vi "FPGA Main.vi"() -> ()   [LabVIEW 2018]
doc: "This FPGA Main VI contains a control loop running in parallel with an RT watchdog loop.\n- The Control Loop performs control calculations on four input channels in parallel, and outputs the results to four output channels.\n- The RT Watchdog Loop checks for a periodic 'pet' from the RT Main VI to ensure communications between RT and FPGA are maintained."
uses:
  controls/Raw Values.ctl
  controls/FPGA State.ctl
  controls/Fill Valves.ctl
  controls/LNG PUGE.ctl
  controls/DECOUPLERS.ctl
  controls/VENT SYSTEM.ctl
  COMET  Extra Programs/controls/TTL Control.ctl
  controls/VENT SYSTEM INDICATORS.ctl
  controls/DECOUPLERS INDICATORS.ctl
  controls/FILL VALVES INDICATORS.ctl
  controls/LOX PURGE.ctl
  controls/LNG PURGE INDICATORS.ctl
  controls/LOX PURGE INDICATORS.ctl
  controls/IN TANK MEASUREMENTS.ctl
  controls/SYSTEM MEASUREMENTS.ctl
  Shared Variables/Flow Controller.ctl
  controls/FM Indicators.ctl
  <vilib>/Platform/TimedLoop/XDataNode/timing_clust.ctl
  <vilib>/Platform/TimedLoop/XDataNode/nitl_modes.ctl
  <vilib>/Platform/TimedLoop/XDataNode/wakeup.ctl
  <vilib>/rvi/FXPMathLib/basic elements/FxpIntAccumulator/subVIs/nifxpmath_IntAccumulator_SimConfig.ctl
  <vilib>/rvi/Emulation/niFpgaGetClockAttributes.vi
  <vilib>/rvi/Emulation/niFpgaSctlEmulationGetInTimedLoop.vi
  <vilib>/rvi/Emulation/niFpgaEmulationReportErrorSimple.vi
  <vilib>/rvi/eio/common/nirviEmuTemplateMethod_errors.vi
  <vilib>/rvi/Analysis/common/codeGenErrors/XNode/niFpgaXNodeCodeGenErrorHandle.vi
  <vilib>/rvi/Emulation/niFpgaCriticalErrorInLSC.vi
  <vilib>/rvi/FXPMathLib/basic elements/FxpIntAccumulator/simVIs/DllFxpIntAccumulator_sub.vi
  <vilib>/rvi/Emulation/niFpgaProcessEmulError.vi
  <vilib>/eio/EIONode/EIONode.xnode
  <vilib>/rvi/Analysis/measure/mean-var-std/XNode/niFpgaMean-Var-Std.xnode
  <vilib>/Platform/TimedLoop/XDataNode/XDataNode.xnode
  <vilib>/rvi/FXPMathLib/basic elements/FxpIntAccumulator/XNode/nifxpmath_IntAccumulator.xnode
  <vilib>/rvi/FXPMathLib/FxpMul/XNode/nifxpmath_Multiplier.xnode
  <vilib>/eio/EIOMethodNode/EIOMethodNode.xnode
  <vilib>/Platform/TimedLoop/XDataNode/XDNodeRunTimeDep.lvlib
  <vilib>/rvi/FXPMathLib/sim/FxpSim.dll
panel:
  out "Flow Controller 2":T1={"LOX_HE_MFC"=0.004, "LNG_HE_MFC"=0.004}
  out "FM Indicators":T2 {"LNG_FMF [GPM]" scale=0.0..10.0; "LOX_FMF [GPM]" scale=0.0..10.0; "LNG_FMP [psi]" scale=0.0..10.0; "LOX_FMP [psi]" scale=0.0..10.0; "LOX_FMT [F]" scale=0.0..100.0; "LNG_FMT [F]" scale=0.0..100.0}
  out "error out 2":errorcluster
  in  "Flow Controller":T1={"LOX_HE_MFC"=0.004, "LNG_HE_MFC"=0.004} {"LNG_HE_MFC" min=0.004 max=0.02 step=1e-06; "LOX_HE_MFC" min=0.004 max=0.02 step=1e-06}
  out "Tick Count(mSec)":u32
  in  "2nd IGN Delay (ms) 2":u32=3000
  in  "Photo 2 Delay (ms)":u32 caption="Count(mSec)"
  out "9401 Fault":bool
  in  "2nd_IGN":bool
  in  "WDW_BRK":bool
  in  "PVC Vent":bool
  out "N2F":sgl format="%#_13g"
  out "Open Current Loop":bool[](array[boolean])
  out "Power Supply Fault":bool
  out "Mod4/AI6/LNG_DST":fxp<+/-,26,5>
  out "9264 Error":bool
  out "error out":errorcluster
  out "SYSTEM MEASUREMENTS":T3 {"LN2 [GPM]" scale=0.004..0.02; "LN2_Temp_Coil" scale=0.0..1.6; "LN2_Temp_HEX" scale=0.0..1.6; "LNG_DST 2" scale=0.004..0.02; "LOX_DST 2" scale=0.004..0.02; "LOX_MSP" scale=0.004..0.02; "LOX_MST" scale=0.004..0.02; "LNG_MSP" scale=0.004..0.02; "LNG_MST" scale=0.0..10.0; "LOX_UST" scale=0.0..10.0; "LNG_UST" scale=0.0..10.0; "LOX_USP" scale=0.0..100.0; "LNG_USP" scale=0.0..10.0; "N2_PURGE [CFM]" scale=0.0..100.0; "LOX_DSP" scale=0.0..10.0; "LOX_DST" scale=0.0..10.0; "LNG_DSP" scale=0.0..100.0; "LNG_DST" scale=0.0..100.0}
  out "IN TANK MEASUREMENTS":T4 {"LNG_TANK_ULEGE 2" scale=0.0..1.0; "LNG_TANK_ULEGE" scale=0.0..5.0; "LOX_TANK_ULEGE 2" scale=0.0..1.0; "LNG_TANK 2" scale=0.0..100.0; "LOX_TANK 2" scale=0.0..100.0; "LOX_DIFF" scale=0.0..100.0; "LNG_DIFF" scale=0.0..100.0; "LOX_TANK_ULEGE" scale=0.0..10.0}
  out "LOX PURGE INDICATORS":T5
  out "LNG PURGE INDICATORS":T6
  in  "LOX PURGE":T7
  out "Fill Valves INDICATORS":T8
  out "DECOUPLERS INDICATORS":T9
  out "VENT SYSTEM INDICATORS":T10
  out "LOX_VCV_FAULT":bool
  out "LNG_VCV_FAULT":bool
  out "LOX_UP":sgl format="%#_13g"
  out "LOX_DIFF":sgl format="%#_13g"
  out "LNG_DIFF":sgl format="%#_13g"
  out "LOX_DSP":sgl format="%#_13g"
  out "LNG_DSP":sgl format="%#_13g"
  out "LOX_DST":sgl format="%#_13g"
  out "LNG_DST":sgl format="%#_13g"
  out "LOX_FMP":sgl format="%#_13g"
  out "LOX_FMT":sgl format="%#_13g"
  out "LNG_FMP":sgl format="%#_13g"
  out "LOX_FMF":sgl format="%#_13g"
  out "LNG_FMT":sgl format="%#_13g"
  out "LNG_FMF":sgl format="%#_13g"
  in  "HP Duration (ms)":u32=2
  in  "Arm":bool
  in  "Manual Ignitor TTL":bool
  in  "Manual Spectrometer TTL":bool
  in  "Manual Camera TTL Secondary":bool
  in  "Manual Camera TTL":bool
  out "x+y 4":u8
  in  "FIRE":bool
  in  "TTL State":T11=enum."OFF"
  in  "Photo Delay (ms)":u32 caption="Count(mSec)"
  in  "VENT SYSTEM":T12
  in  "DECOUPLERS":T13
  in  "LNG PURGE":T14
  in  "Fill Valves":T15 {"LOX_VCV_CTL" scale=0.004..0.02 scale format="%.2f"; "LNG_VCV_CTL" scale=0.004..0.02 scale format="%.6f"}
  out "9265 Error":bool
  out "Input Error":bool
  out "Current FPGA State":T16=enum."Manual"
  in  "Control Period (ticks)":u32
  out "Actual Loop Period (ticks)":u32
  in  "Change State":bool
  in  "New State":T16=enum."Control"
  out "VALVE POS":T17 {"LOX_VCV_POS" scale=0.0..10.0; "LNG_VCV_POS" scale=0.0..10.0}
  out "Watchdog Timed Out?":bool=TRUE
  in  "Enable Watchdog":bool
  in  "Pet Watchdog":bool
  in  "Watchdog Timeout Period (ticks)":u64=40000000 format="%.0p"
  out "Time Since Last Pet":u64
  # "Watchdog Settings"
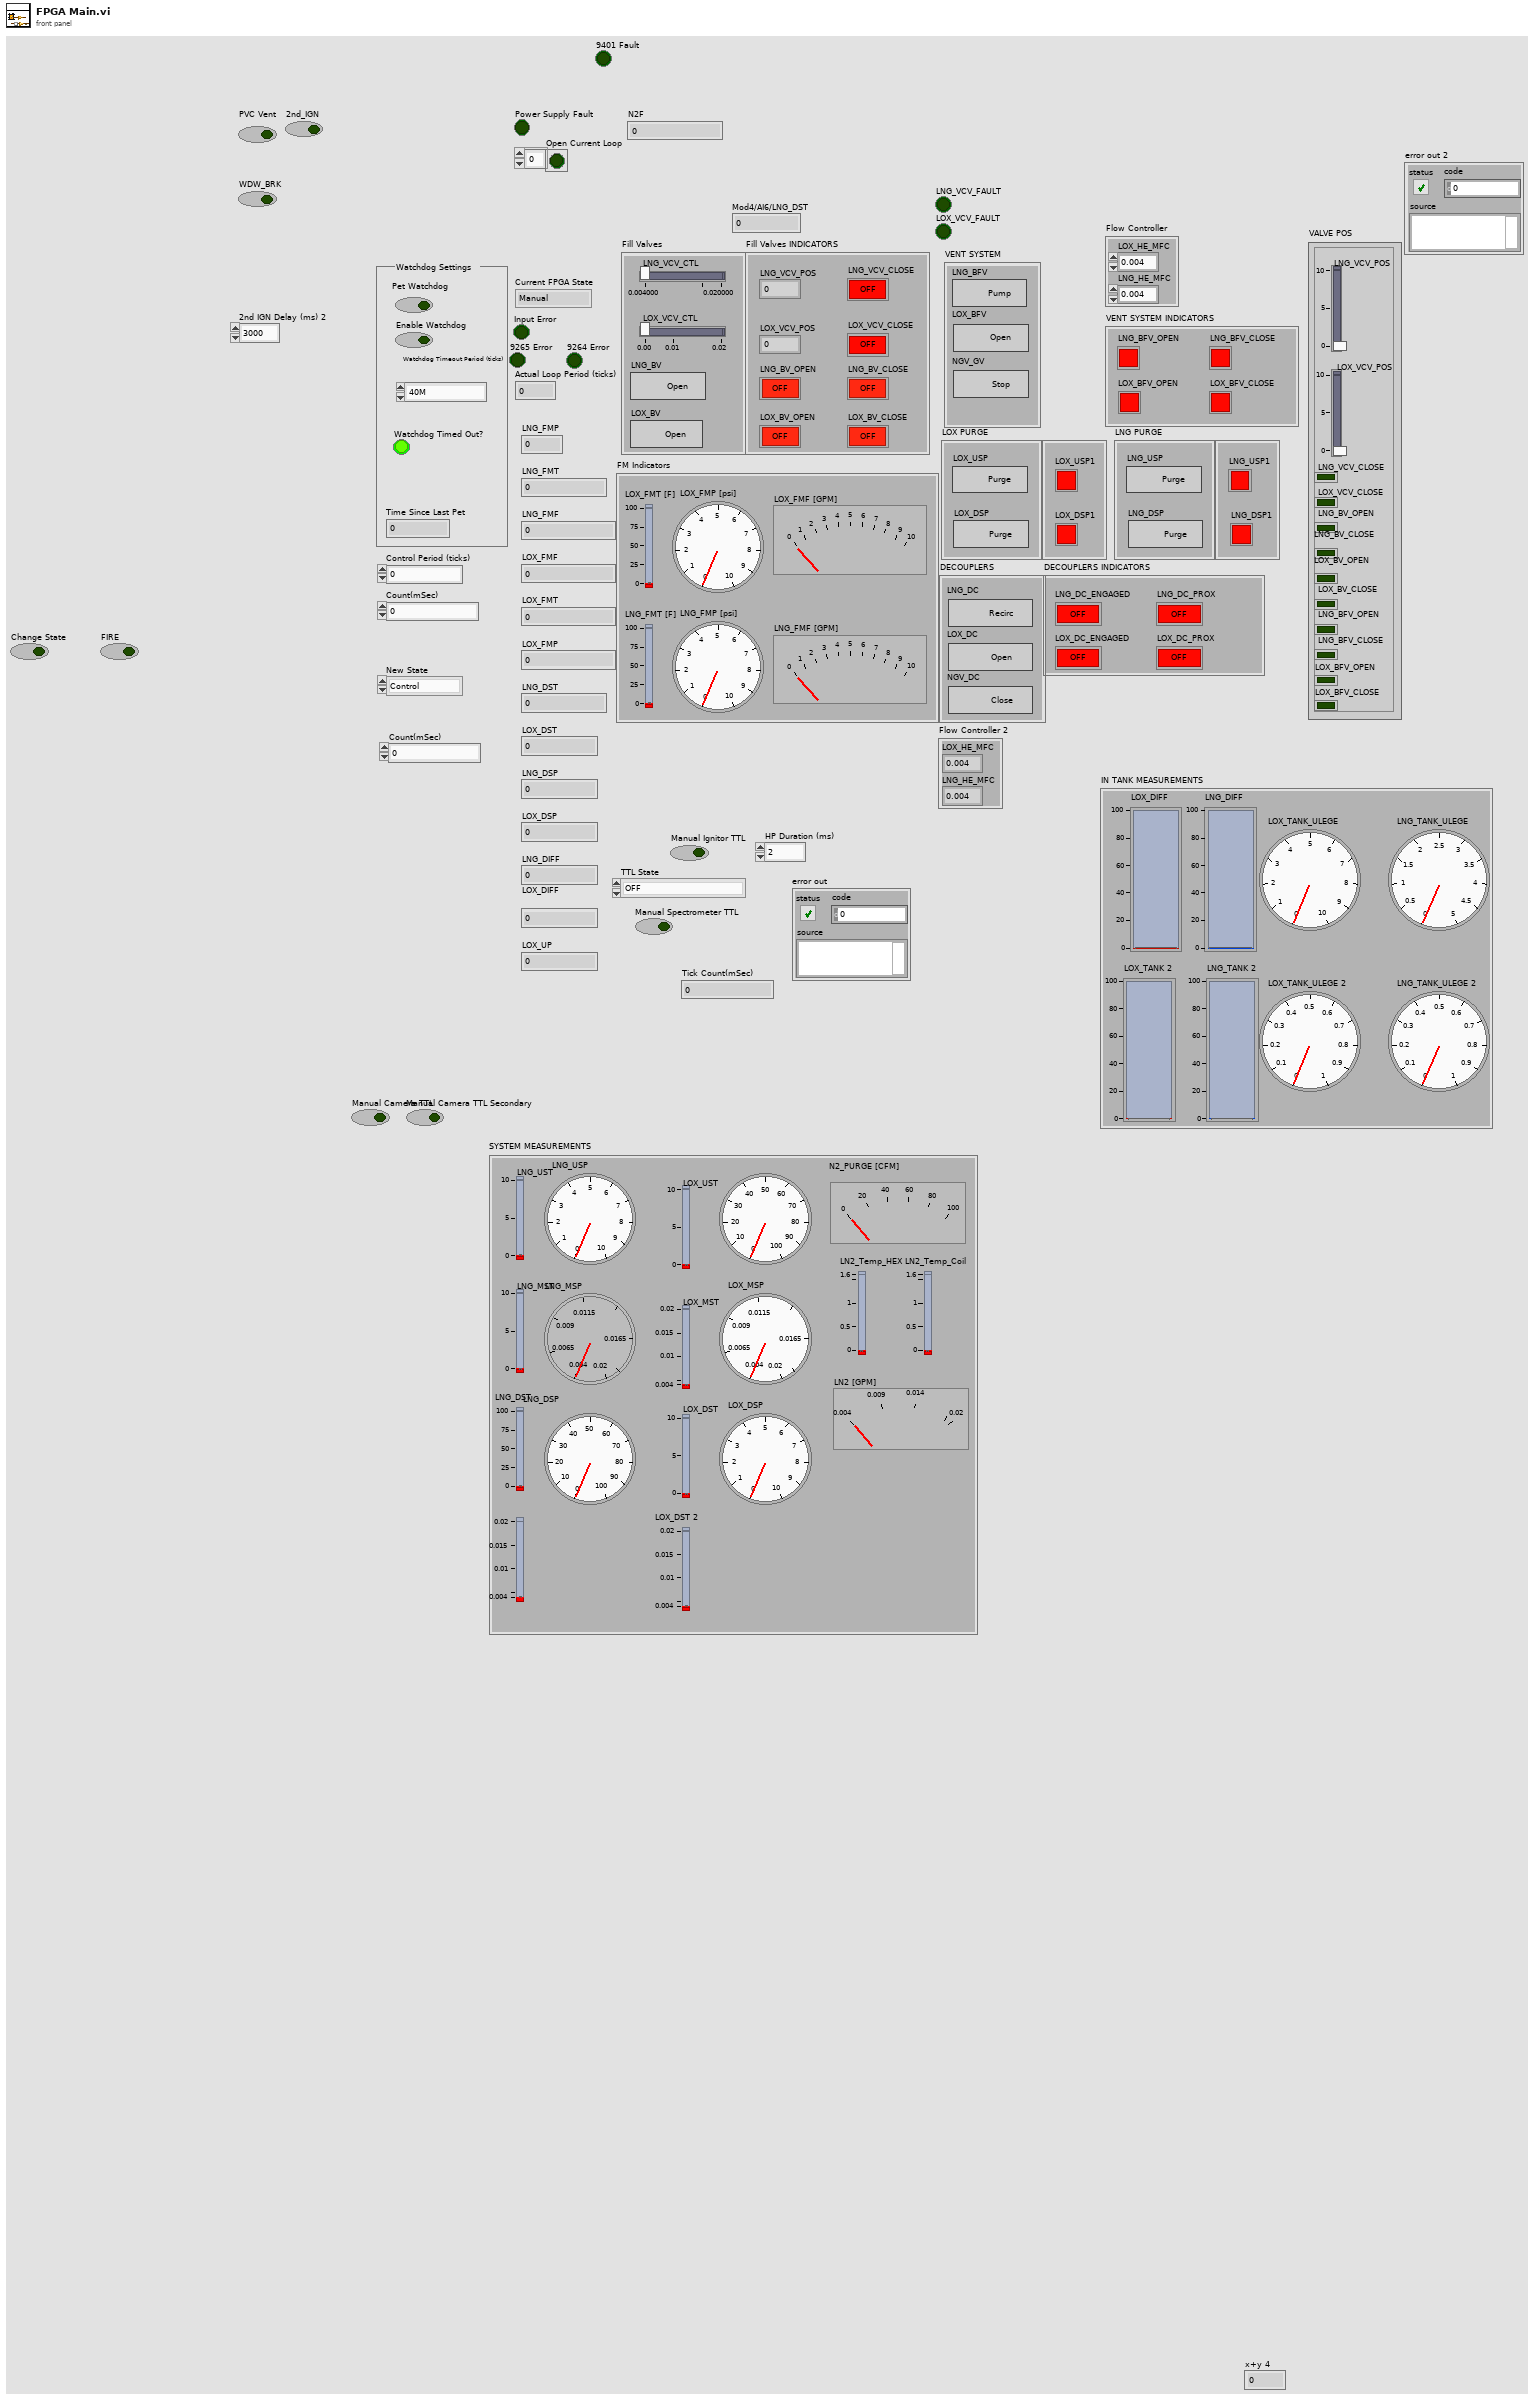
[diagram p1: front panel]
types:
  T1 = typedef "Flow Controller.ctl" = cluster{"LOX_HE_MFC":sgl, "LNG_HE_MFC":sgl}
  T2 = typedef "FM Indicators.ctl" = cluster{"LNG_FMT [F]":sgl, "LOX_FMT [F]":sgl, "LOX_FMP [psi]":sgl, "LNG_FMP [psi]":sgl, "LOX_FMF [GPM]":sgl, "LNG_FMF [GPM]":sgl}
  T3 = typedef "SYSTEM MEASUREMENTS.ctl" = cluster{"LNG_DST":sgl, "LNG_DSP":sgl, "LOX_DST":sgl, "LOX_DSP":sgl, "N2_PURGE [CFM]":sgl, "LNG_USP":sgl, "LOX_USP ":sgl, "LNG_UST":sgl, "LOX_UST":sgl, "LNG_MST":sgl, "LNG_MSP":sgl, "LOX_MST\n":sgl, "LOX_MSP":sgl, "LOX_DST 2":sgl, "LNG_DST 2":sgl, "LN2_Temp_HEX":sgl, "LN2_Temp_Coil":sgl, "LN2 [GPM]":sgl}
  T4 = typedef "IN TANK MEASUREMENTS.ctl" = cluster{"LOX_TANK_ULEGE":sgl, "LNG_DIFF":sgl, "LOX_DIFF":sgl, "LOX_TANK 2":sgl, "LNG_TANK 2":sgl, "LOX_TANK_ULEGE 2":sgl, "LNG_TANK_ULEGE":sgl, "LNG_TANK_ULEGE 2":sgl}
  T5 = typedef "LOX PURGE INDICATORS.ctl" = cluster{"LOX_USP1":bool, "LOX_DSP1":bool}
  T6 = typedef "LNG PURGE INDICATORS.ctl" = cluster{"LNG_USP1":bool, "LNG_DSP1":bool}
  T7 = typedef "LOX PURGE.ctl" = cluster{"LOX_USP":bool, "LOX_DSP":bool}
  T8 = typedef "FILL VALVES INDICATORS.ctl" = cluster{"LNG_BV_CLOSE":bool, "LOX_BV_CLOSE":bool, "LNG_VCV_CLOSE":bool, "LNG_VCV_POS":sgl, "LOX_VCV_POS":sgl, "LNG_BV_OPEN":bool, "LOX_BV_OPEN":bool, "LOX_VCV_CLOSE":bool}
  T9 = typedef "DECOUPLERS INDICATORS.ctl" = cluster{"LNG_DC_ENGAGED":bool, "LOX_DC_ENGAGED":bool, "LNG_DC_PROX":bool, "LOX_DC_PROX":bool}
  T10 = typedef "VENT SYSTEM INDICATORS.ctl" = cluster{"LNG_BFV_CLOSE":bool, "LOX_BFV_CLOSE":bool, "LNG_BFV_OPEN":bool, "LOX_BFV_OPEN":bool}
  T11 = typedef "TTL Control.ctl" = enum16{"AUTO", "MANUAL", "OFF"}
  T12 = typedef "VENT SYSTEM.ctl" = cluster{"LNG_BFV":bool, "LOX_BFV":bool, "NGV_GV":bool}
  T13 = typedef "DECOUPLERS.ctl" = cluster{"LNG_DC":bool, "LOX_DC":bool, "NGV_DC":bool}
  T14 = typedef "LNG PUGE.ctl" = cluster{"LNG_USP":bool, "LNG_DSP":bool}
  T15 = typedef "Fill Valves.ctl" = cluster{"LOX_BV":bool, "LNG_BV":bool, "LNG_VCV_CTL":sgl, "LOX_VCV_CTL":sgl}
  T16 = typedef "FPGA State.ctl" = enum16{"Safe State", "Manual", "Control"}
  T17 = typedef "Raw Values.ctl" = cluster{"LNG_VCV_POS":i16, " LOX_VCV_POS":i16, "LNG_VCV_CLOSE":bool, "LOX_VCV_CLOSE":bool, "LNG_BV_OPEN":bool, "LNG_BV_CLOSE":bool, "LOX_BV_OPEN":bool, "LOX_BV_CLOSE":bool, "LNG_BFV_OPEN":bool, "LNG_BFV_CLOSE":bool, "LOX_BFV_OPEN":bool, "LOX_BFV_CLOSE":bool}
  T18 = typedef "XDNodeRunTimeDep.lvlib/timing_clust.ctl" = cluster{"Expected End [f-1]":u64, "Actual End [f-1]":u64, "Finished Late? [f-1]":bool, "Expected End [i-1]":u64, "Actual End [i-1]":u64, "Finished Late? [i-1]":bool, "Expected Start [i]":u64, "Actual Start [i]":u64, "Expected Start [f]":u64, "Actual Start [f]":u64, "Source Name":string, "Structure Name":string, "Period":i64, "Deadline":i64, "Offset":i64, "Start":i64, "Priority":i32, "Timeout":i32, "Mode":T19, "Wakeup Reason":T20, "Error":errorcluster, "Source Type":string, "Secondary Source Type":string, "Global End Time":u64, "Global Start Time":u64, "Frame Duration":u64, "Iteration Duration":u64, "Assigned CPU":i32, "I/O Scan Engine Mode":u32}
  T19 = typedef "XDNodeRunTimeDep.lvlib/nitl_modes.ctl" = enum32{"No Change", "Process missed periods, maintain original phase", "Discard missed periods, maintain original phase", "Process missed periods, ignore original phase", "Discard missed periods, ignore original phase"}
  T20 = typedef "XDNodeRunTimeDep.lvlib/wakeup.ctl" = enum32{"Normal", "Aborted", "Asynchronous wakeup", "Timing source error", "Timed loop error", "Timeout"}
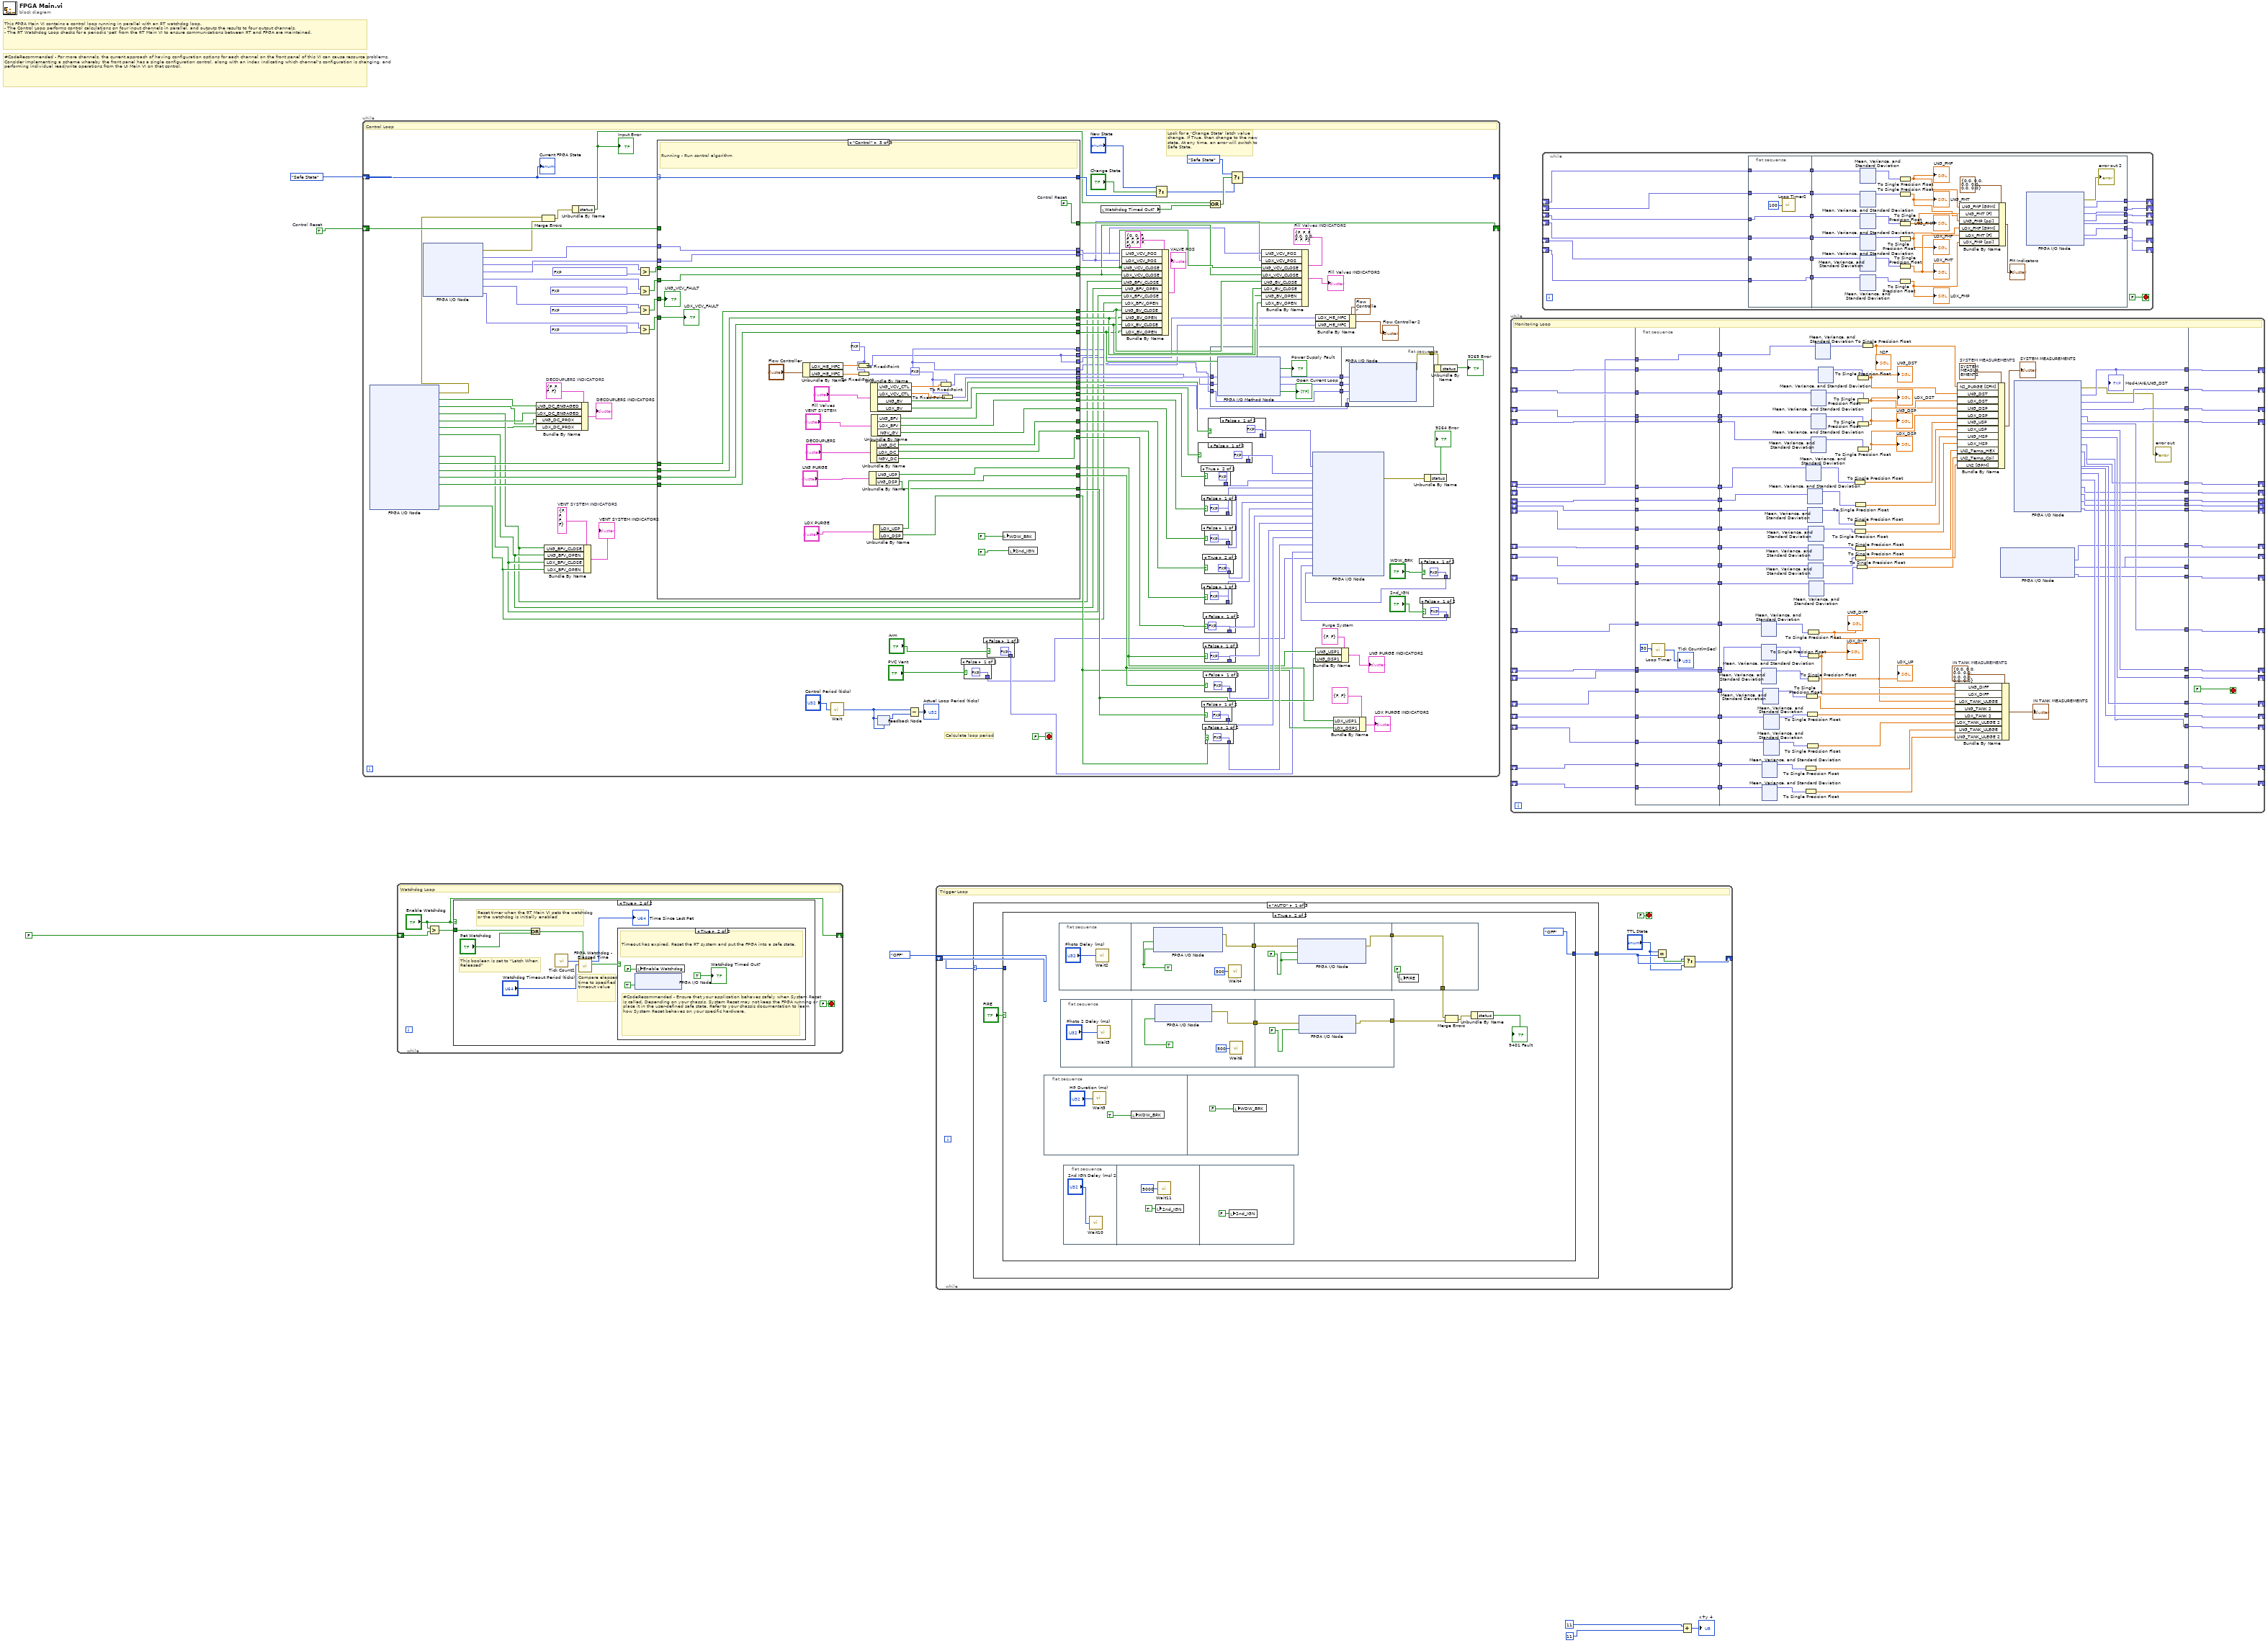
[diagram p0: block diagram]
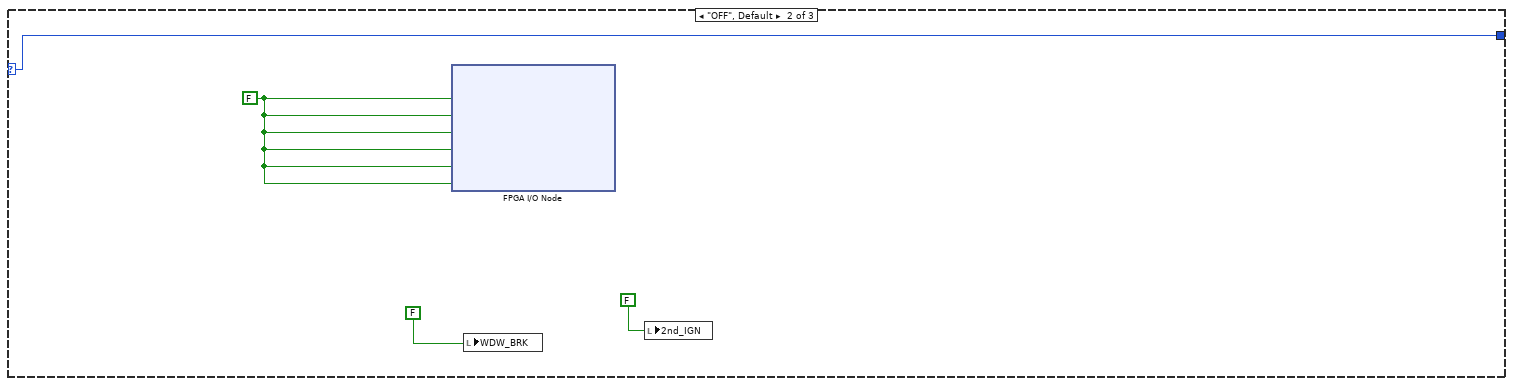
[diagram p3: hidden frame]
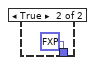
[diagram p5: hidden frame]
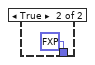
[diagram p6: hidden frame]
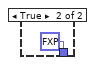
[diagram p7: hidden frame]
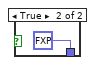
[diagram p8: hidden frame]
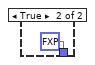
[diagram p9: hidden frame]
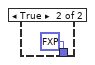
[diagram p10: hidden frame]
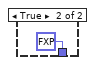
[diagram p11: hidden frame]
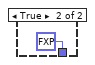
[diagram p12: hidden frame]
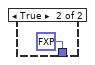
[diagram p13: hidden frame]
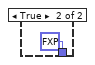
[diagram p14: hidden frame]
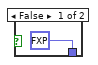
[diagram p15: hidden frame]
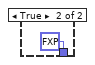
[diagram p16: hidden frame]
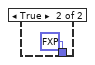
[diagram p17: hidden frame]
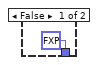
[diagram p18: hidden frame]
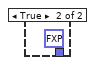
[diagram p19: hidden frame]
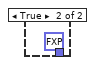
[diagram p20: hidden frame]
diagram:
  w6 = TRUE  # Control Reset
  # "#CodeRecommended - For more channels, the current approach of having configuration options for each channel on the front panel of this VI can cause resource problems.  Consider implementing a scheme whereby the front panel has a single configuration control, along with an index indicating which channel's configuration is changing, and performing individual read/write operations from the UI Main VI on that control."
  # "This FPGA Main VI contains a control loop running in parallel with an RT watchdog loop.\n- The Control Loop performs control calculations on four input channels in parallel, and outputs the results to four output channels.\n- The RT Watchdog Loop checks for a periodic 'pet' from the RT Main VI to ensure communications between RT and FPGA are maintained."
  n1 = while {
    shift-right: [w117] -> _
    shift-left: FPGA_State."Safe State" ("FPGA State") -> [w102]
    shift-right: [w114] -> _
    shift-left: w6 -> [w113]
    stop <- FALSE stop-if-true
    w60 = T8 {"LNG_BV_CLOSE"=FALSE, "LOX_BV_CLOSE"=FALSE, "LNG_VCV_CLOSE"=FALSE, "LNG_VCV_POS"=0.0, "LOX_VCV_POS"=0.0, "LNG_BV_OPEN"=FALSE, "LOX_BV_OPEN"=FALSE, "LOX_VCV_CLOSE"=FALSE}  # Fill Valves INDICATORS
    w52 = T6 {"LNG_USP1"=FALSE, "LNG_DSP1"=FALSE}  # Purge System
    w67 = T9 {"LNG_DC_ENGAGED"=FALSE, "LOX_DC_ENGAGED"=FALSE, "LNG_DC_PROX"=FALSE, "LOX_DC_PROX"=FALSE}  # DECOUPLERS INDICATORS
    w64 = T10 {"LNG_BFV_CLOSE"=FALSE, "LOX_BFV_CLOSE"=FALSE, "LNG_BFV_OPEN"=FALSE, "LOX_BFV_OPEN"=FALSE}  # VENT SYSTEM INDICATORS
    # "Calculate loop period"
    # "Look for a 'Change State' latch value change. If True, then change to the new state. At any time, an error will switch to Safe State."
    # "Control Loop"
    n2 = xnode "FPGA I/O Node"() -> ("error out"=w78:errorcluster, "ZS-02 (LNG_DC_LIMIT)"=w66:bool, "XY-02 (LNG_DC_PROX)"=w15:bool, "XAL-02 (LNG_BFV)"=w26:bool, "ZS-01 (LOX_DC_LIMIT)"=w65:bool, "XY-01 (LOX_DC_PROX)"=w14:bool, "XAH-02 (LNG_BFV)"=w27:bool, "XAL-01 (LOX_BFV)"=w28:bool, "XAL_04 (LNG_BV)"=w61:bool, "XAH-04 (LNG_BV)"=w62:bool, "XAL-13 (LOX_BV)"=w57:bool, "XAH-13 (LOX_BV)"=w63:bool, "XAH-01 (LOX_BFV)"=w29:bool)  [unwired: 17 in, 20 out]
    n3 = xnode "FPGA I/O Node"() -> ("error out"=w77:errorcluster, "XY-04 (LNG_VCV)"=w88:fxp<+/-,24,-4>, "XAL-07 (LNG_VCV)"=w10:fxp<+/-,24,-4>, "XY-03 (LOX_VCV)"=w87:fxp<+/-,24,-4>, "XAL-12 (LOX_VCV)"=w11:fxp<+/-,24,-4>, "ZA-02 (LNG_VCV)"=w13:fxp<+/-,24,-4>, "ZA-01 (LOX_VCV)"=w12:fxp<+/-,24,-4>)  [unwired: 7 in, 6 out]
    n4 = Bundle By Name(cluster=w67, "LNG_DC_ENGAGED"=w66, "LOX_DC_ENGAGED"=w65, "LNG_DC_PROX"=w15, "LOX_DC_PROX"=w14) -> (→"DECOUPLERS INDICATORS":T9)
    n5 = Merge Errors(w78, w77) -> (w76:errorcluster)
    n6 = Bundle By Name(cluster=w64, "LNG_BFV_CLOSE"=w26, "LNG_BFV_OPEN"=w27, "LOX_BFV_CLOSE"=w28, "LOX_BFV_OPEN"=w29) -> (→"VENT SYSTEM INDICATORS":T10)
    n7 = Unbundle By Name(w76) -> ("status"=w109:bool)
    "Input Error" <- w109
    n8 = Greater?(x=w10, y=fxp<+/-,24,-4> 0.0040000006556510925) -> (0:w85:bool)
    n9 = Greater?(x=w11, y=fxp<+/-,24,-4> 0.006000000983476639) -> (0:w81:bool)
    n10 = Greater?(x=w13, y=fxp<+/-,24,-4> 0.006000000983476639) -> (0:w80:bool)
    n11 = Greater?(x=w12, y=fxp<+/-,24,-4> 0.006000000983476639) -> (0:w79:bool)
    n12 = case shown="\"Control\"" w102 {
      selector: w102 -> [w176 w195 w237]
      tunnel: [w176 w195 w237] -> w112
      tunnel: [w177 w196 w238] -> w114
      tunnel: w113 -> [_ _ _]
      tunnel: [w174 w188 w221] -> w9
      tunnel: [w164 w194 w228] -> w99
      tunnel: [w164 w194 w227] -> w98
      tunnel: [w164 w194 w226] -> w97
      tunnel: [w164 w194 w225] -> w94
      tunnel: [w164 w194 w224] -> w92
      tunnel: [w164 w194 w232] -> w90
      tunnel: [w164 w194 w231] -> w74
      tunnel: [w164 w194 w230] -> w89
      tunnel: [w164 w194 w229] -> w51
      tunnel: [w164 w189 w208] -> w43
      tunnel: [w173 w187 w220] -> w8
      tunnel: [w164 w189 w207] -> w50
      tunnel: w88 -> [w174 w188 w221]
      tunnel: w87 -> [w173 w187 w220]
      tunnel: w85 -> [w172 w186 w219]
      tunnel: w81 -> [w171 w185 w218]
      tunnel: w80 -> [w170 w184 w213]
      tunnel: w79 -> [w169 w183 w212]
      tunnel: [w172 w186 w219] -> w59
      tunnel: [w171 w185 w218] -> w58
      tunnel: [w168 w182 w217] -> w56
      tunnel: w61 -> [w168 w182 w217]
      tunnel: [w167 w181 w216] -> w54
      tunnel: w62 -> [w167 w181 w216]
      tunnel: [w166 w180 w215] -> w55
      tunnel: w57 -> [w166 w180 w215]
      tunnel: [w165 w179 w214] -> w53
      tunnel: w63 -> [w165 w179 w214]
      tunnel: [w164 w189 w210] -> w42
      tunnel: [w163 w178 w204] -> w39
      tunnel: [w163 w178 w209] -> w38
      tunnel: [w163 w178 w199] -> w18
      tunnel: [w163 w178 w198] -> w19
      tunnel: [w163 w178 w198] -> w17
      tunnel: [w163 w178 w199] -> w16
      frame "Safe State", Default {
        (unwired) sgl 0.0 ("LNG_HE_MFC")
        w163 = fxp<+,20,-5> 0.0 ("AO 3")
        w164 = FALSE ("Watchdog Timed Out?")
        w177 = TRUE  # Control Reset
        # "'Safe State' runs on FPGA startup.  This loop does not move into the 'Manual' or 'Running' state until directed by the Real-Time target. If an I/O error occurs on the FPGA, or if the RT watchdog times out, this loop will move back into 'Safe State'."
        # "Reset Watchdog Timed Out flag in case that's what got the control loop into the Safe State in the first place."
        n13 = local write "LNG_VCV_FAULT"(w170) -> ()
        n14 = local write "LOX_VCV_FAULT"(w169) -> ()
        n15 = local write "Watchdog Timed Out?"(FALSE ("Watchdog Timed Out?")) -> ()
      }
      frame "Manual" {
        (unwired) sgl 0.0 ("LNG_HE_MFC")
        w178 = fxp<+,20,-5> 0.0 ("AO 3")
        w189 = FALSE
        w194 = FALSE
        w196 = TRUE  # Control Reset
        # "Manual - Specify output values based on values from UI Main VI"
        n16 = local write "LNG_VCV_FAULT"(w184) -> ()
        n17 = local write "LOX_VCV_FAULT"(w183) -> ()
        n18 = xnode "FPGA I/O Node"("Spectrometer TTL"="Manual Spectrometer TTL", "Camera TTL"="Manual Camera TTL", "Secondary Camera TTL"="Manual Camera TTL Secondary", "Ignitor"="Manual Ignitor TTL") -> ()  [unwired: 5 in, 5 out]
        n19 = xnode "FPGA I/O Node"("Mod5/DO15"="Manual Ignitor TTL") -> ()  [unwired: 2 in, 2 out]
      }
      frame "Control" {
        w197 = fxp<+,1,1> 0.0
        w203 = fxp<+,20,-5> 0.0 ("AO 3")
        w238 = FALSE  # Control Reset
        # "Running - Run control algorithm"
        n20 = Unbundle By Name("Flow Controller") -> ("LOX_HE_MFC"=w200:sgl, "LNG_HE_MFC"=w201:sgl)
        n21 = To Fixed-Point(fixed-point type=w197, number=w200) -> (fixed-point=w198:fxp<+,1,1>)
        n22 = To Fixed-Point(fixed-point type=w197, number=w201) -> (fixed-point=w199:fxp<+,1,1>)
        n23 = Unbundle By Name("LNG PURGE") -> ("LNG_USP"=w229:bool, "LNG_DSP"=w207:bool)
        n24 = Unbundle By Name("DECOUPLERS") -> ("LNG_DC"=w232:bool, "LOX_DC"=w231:bool, "NGV_DC"=w230:bool)
        n25 = Unbundle By Name("Fill Valves") -> ("LNG_VCV_CTL"=w222:sgl, "LOX_VCV_CTL"=w223:sgl, "LNG_BV"=w228:bool, "LOX_BV"=w227:bool)
        n26 = Unbundle By Name("VENT SYSTEM") -> ("LNG_BFV"=w226:bool, "LOX_BFV"=w225:bool, "NGV_GV"=w224:bool)
        n27 = Unbundle By Name("LOX PURGE") -> ("LOX_USP"=w208:bool, "LOX_DSP"=w210:bool)
        n28 = To Fixed-Point(fixed-point type=w203, number=w222) -> (fixed-point=w204:fxp<+,20,-5>)
        n29 = To Fixed-Point(fixed-point type=w203, number=w223) -> (fixed-point=w209:fxp<+,20,-5>)
        n30 = local write "WDW_BRK"(FALSE) -> ()
        n31 = local write "2nd_IGN"(FALSE ("2nd_IGN")) -> ()
        "LNG_VCV_FAULT" <- w213
        "LOX_VCV_FAULT" <- w212
      }
    }
    n32 = call "Wait"("Count(Ticks)"="Control Period (ticks)") -> ("Tick Count(Ticks)"=w106:u32)
    n33 = feedback-in #1(w106) -> ()
    n34 = feedback #1(w106) -> (w105:u32)
    n35 = Subtract(x=w106, y=w105) -> (x-y=→"Actual Loop Period (ticks)":u32)
    n36 = case shown="False" "PVC Vent" {
      tunnel: [fxp<+/-,20,5> 0.0 ("N2_FILL_VALVE_2") fxp<+/-,20,5> 5.0 ("N2_FILL_VALVE_2")] -> w33
      frame False {
      }
      frame True {
      }
    }
    n37 = case shown="False" "Arm" {
      tunnel: [fxp<+/-,20,5> 5.0 ("N2_FILL_VALVE_2") fxp<+/-,20,5> 0.0 ("N2_FILL_VALVE_2")] -> w34
      frame False {
      }
      frame True {
      }
    }
    n38 = local read "Watchdog Timed Out?"() -> (w107:bool)
    n39 = Bundle By Name(cluster=T17 {"LNG_VCV_POS"=0, " LOX_VCV_POS"=0, "LNG_VCV_CLOSE"=FALSE, "LOX_VCV_CLOSE"=FALSE, "LNG_BV_OPEN"=FALSE, "LNG_BV_CLOSE"=FALSE, "LOX_BV_OPEN"=FALSE, "LOX_BV_CLOSE"=FALSE, "LNG_BFV_OPEN"=FALSE, "LNG_BFV_CLOSE"=FALSE, "LOX_BFV_OPEN"=FALSE, "LOX_BFV_CLOSE"=FALSE} ("Raw Values"), "LNG_VCV_POS"=w9, "LOX_VCV_POS"=w8, "LNG_VCV_CLOSE"=w59, "LOX_VCV_CLOSE"=w58, "LNG_BFV_CLOSE"=w26, "LNG_BFV_OPEN"=w27, "LOX_BFV_CLOSE"=w28, "LOX_BFV_OPEN"=w29, "LNG_BV_CLOSE"=w56, "LNG_BV_OPEN"=w54, "LOX_BV_CLOSE"=w55, "LOX_BV_OPEN"=w53) -> (→"VALVE POS":T17)
    n40 = Select(t="New State", s="Change State", f=w112) -> (s? t:f=w110:T16)
    n41 = case shown="False" w98 {
      tunnel: [fxp<+/-,20,5> 0.0 ("N2_FILL_VALVE_2") fxp<+/-,20,5> 5.0 ("N2_FILL_VALVE_2")] -> w96
      frame False {
      }
      frame True {
      }
    }
    n42 = case shown="True" w97 {
      tunnel: [fxp<+/-,20,5> 0.0 ("N2_FILL_VALVE_2") fxp<+/-,20,5> 5.0 ("N2_FILL_VALVE_2")] -> w95
      frame False {
      }
      frame True {
      }
    }
    n43 = case shown="False" w94 {
      tunnel: [fxp<+/-,20,5> 0.0 ("N2_FILL_VALVE_2") fxp<+/-,20,5> 5.0 ("N2_FILL_VALVE_2")] -> w93
      frame False {
      }
      frame True {
      }
    }
    n44 = case shown="False" w92 {
      tunnel: [fxp<+/-,20,5> 0.0 ("N2_FILL_VALVE_2") fxp<+/-,20,5> 5.0 ("N2_FILL_VALVE_2")] -> w91
      frame False {
      }
      frame True {
      }
    }
    n45 = case shown="True" w90 {
      tunnel: [fxp<+/-,20,5> 0.0 ("N2_FILL_VALVE_2") fxp<+/-,20,5> 5.0 ("N2_FILL_VALVE_2")] -> w75
      frame False {
      }
      frame True {
      }
    }
    n46 = case shown="False" w74 {
      tunnel: [fxp<+/-,20,5> 0.0 ("N2_FILL_VALVE_2") fxp<+/-,20,5> 5.0 ("N2_FILL_VALVE_2")] -> w73
      frame False {
      }
      frame True {
      }
    }
    n47 = case shown="False" w89 {
      tunnel: [fxp<+/-,20,5> 0.0 ("N2_FILL_VALVE_2") fxp<+/-,20,5> 5.0 ("N2_FILL_VALVE_2")] -> w72
      frame False {
      }
      frame True {
      }
    }
    n48 = case shown="False" w51 {
      tunnel: [fxp<+/-,20,5> 0.0 ("N2_FILL_VALVE_2") fxp<+/-,20,5> 5.0 ("N2_FILL_VALVE_2")] -> w71
      frame False {
      }
      frame True {
      }
    }
    n49 = case shown="False" w43 {
      tunnel: [fxp<+/-,20,5> 0.0 ("N2_FILL_VALVE_2") fxp<+/-,20,5> 5.0 ("N2_FILL_VALVE_2")] -> w70
      frame False {
      }
      frame True {
      }
    }
    n50 = case shown="False" w50 {
      tunnel: [fxp<+/-,20,5> 0.0 ("N2_FILL_VALVE_2") fxp<+/-,20,5> 5.0 ("N2_FILL_VALVE_2")] -> w69
      frame False {
      }
      frame True {
      }
    }
    n51 = case shown="False" w42 {
      tunnel: [fxp<+/-,20,5> 0.0 ("N2_FILL_VALVE_2") fxp<+/-,20,5> 5.0 ("N2_FILL_VALVE_2")] -> w68
      frame False {
      }
      frame True {
      }
    }
    n52 = case shown="False" w99 {
      tunnel: [fxp<+/-,20,5> 0.0 ("N2_FILL_VALVE_2") fxp<+/-,20,5> 5.0 ("N2_FILL_VALVE_2")] -> w22
      frame False {
      }
      frame True {
      }
    }
    n53 = flat-sequence {
      tunnel: w38 -> [w132]
      tunnel: w39 -> [w133]
      tunnel: [w133] -> w37
      tunnel: [w132] -> w36
      tunnel: w16 -> [w129]
      tunnel: [w129] -> w23
      tunnel: [w138] -> w119
      tunnel: w37 -> [w134]
      tunnel: w36 -> [w135]
      tunnel: w23 -> [w136]
      tunnel: w17 -> [w137]
      frame #0 {
        n54 = xnode "FPGA I/O Method Node"() -> ("Power Supply Fault"=→"Power Supply Fault":bool, "Open Current Loop"=→"Open Current Loop":bool[])  [unwired: 2 in, 2 out]
      }
      frame #1 {
        n55 = xnode "FPGA I/O Node"("CV-02 (LNG_VCV)"=w134, "CV-01 (LOX_VCV)"=w135, "FC-05 (LNG_HE_MFC)"=w136, "FC-04 (LOX_HE_MFC)"=w137) -> ("error out"=w138:errorcluster)  [unwired: 5 in, 4 out]
      }
    }
    n56 = Compound Arithmetic op=OR(w109, w107) -> (w116:bool)
    n57 = Select(t=FPGA_State."Safe State" ("FPGA State"), s=w116, f=w110) -> (s? t:f=w117:T16)
    n58 = Bundle By Name(cluster=w60, "LNG_VCV_POS"=w9, "LOX_VCV_POS"=w8, "LNG_VCV_CLOSE"=w59, "LOX_VCV_CLOSE"=w58, "LNG_BV_CLOSE"=w56, "LOX_BV_CLOSE"=w55, "LNG_BV_OPEN"=w54, "LOX_BV_OPEN"=w53) -> (→"Fill Valves INDICATORS":T8)
    n59 = Bundle By Name(cluster=T1 {"LOX_HE_MFC"=0.004, "LNG_HE_MFC"=0.004} ("Flow Controller 2"), "LOX_HE_MFC"=w19, "LNG_HE_MFC"=w18) -> (→"Flow Controller 2":T1)
    n60 = Bundle By Name(cluster=w52, "LNG_USP1"=w51, "LNG_DSP1"=w50) -> (→"LNG PURGE INDICATORS":T6)
    n61 = Bundle By Name(cluster=T5 {"LOX_USP1"=FALSE, "LOX_DSP1"=FALSE} ("Purge System"), "LOX_USP1"=w43, "LOX_DSP1"=w42) -> (→"LOX PURGE INDICATORS":T5)
    n62 = case shown="False" "WDW_BRK" {
      tunnel: [fxp<+/-,20,5> 0.0 ("N2_FILL_VALVE_2") fxp<+/-,20,5> 5.0 ("N2_FILL_VALVE_2")] -> w31
      frame False {
      }
      frame True {
      }
    }
    n63 = case shown="False" "2nd_IGN" {
      tunnel: [fxp<+/-,20,5> 0.0 ("N2_FILL_VALVE_2") fxp<+/-,20,5> 5.0 ("N2_FILL_VALVE_2")] -> w30
      frame False {
      }
      frame True {
      }
    }
    n64 = xnode "FPGA I/O Node"("Mod6/AO0/LNG_BV"=w22, "Mod6/AO1/LOX_BV"=w96, "Mod6/AO2/LNG_BFV"=w95, "Mod6/AO3/LOX_BFV"=w93, "Mod6/AO4/NGV_GV"=w91, "Mod6/AO5/LNG_DC"=w75, "Mod6/AO6/LOX_DC"=w73, "Mod6/AO7/NGV_DC"=w72, "Mod6/AO8/LNG_USP"=w71, "Mod6/AO9/LOX_USP"=w70, "Mod6/AO10/LNG_DSP"=w69, "Mod6/AO11/LOX_DSP"=w68, "Mod6/AO12/HP"=w34, "Mod6/AO15/PVC_Vent"=w33, "Mod6/AO13/2nd_IGN"=w30, "Mod6/AO14/WDW_BRK"=w31) -> ("error out"=w41:errorcluster)  [unwired: 17 in, 16 out]
    n65 = Unbundle By Name(w41) -> ("status"=→"9264 Error":bool)
    n66 = Unbundle By Name(w119) -> ("status"=→"9265 Error":bool)
    "Current FPGA State" <- w102
  }
  n67 = while "RT Watchdog Loop" {
    shift-right: ["Enable Watchdog"] -> _
    shift-left: FALSE ("Enable RT Watchdog") -> [w242]
    stop <- FALSE stop-if-true
    # "Watchdog Loop"
    n68 = Greater?(x="Enable Watchdog", y=w242) -> (0:w239:bool)
    n69 = case shown="True" "Enable Watchdog" {
      tunnel: w239 -> [_ w245]
      frame False {
        # "This loop has to be explicitly enabled from the RT Main VI.  This reduces the possiblity of an endless reboot cycle."
      }
      frame True {
        # "This boolean is set to \"Latch When Released\""
        # "Compare elapsed time to specified timeout value"
        # "Reset timer when the RT Main VI pets the watchdog or the watchdog is initially enabled"
        n70 = Or(x=w245, y="Pet Watchdog") -> (x .or. y?=w244:bool)
        n71 = call "Tick Count2"() -> ("Tick Count(Ticks)"=w248:u32)
        n72 = call "FPGA Watchdog - Elapsed Time.vi"("Reset"=w244, "Timeout Period"="Watchdog Timeout Period (ticks)", "Current Time"=w248) -> ("Timeout"=w243:bool, "Elapsed Time"=→"Time Since Last Pet":u64)  [unwired: 7 in]
        n73 = case shown="True" w243 {
          frame False {
            # "Timeout has not expired."
          }
          frame True {
            # "#CodeRecommended - Ensure that your application behaves safely when System Reset is called. Depending on your chassis, System Reset may not keep the FPGA running or place it in the user-defined safe state. Refer to your chassis documentation to learn how System Reset behaves on your specific hardware."
            # "Timeout has expired. Reset the RT system and put the FPGA into a safe state."
            n74 = xnode "FPGA I/O Node"("System Reset"=TRUE ("RT Reset on Watchdog Failure?")) -> ()  [unwired: 1 in, 1 out]
            n75 = local write "Enable Watchdog"(FALSE ("Enable RT Watchdog")) -> ()
            "Watchdog Timed Out?" <- TRUE ("Watchdog Timed Out?")
          }
        }
      }
    }
  }
  n76 = while "RT Watchdog Loop" {
    shift-right: [w254] -> _
    shift-left: TTL_Control."OFF" ("TTL State") -> [w253]
    stop <- FALSE stop-if-true
    # "Trigger Loop"
    n77 = case shown="\"AUTO\"" w253 {
      selector: w253 -> [w260 w297 w298]
      tunnel: [w259 w297 w298] -> w256
      frame "AUTO" {
        n78 = case shown="True" "FIRE" {
          tunnel: w260 -> [w262 _]
          tunnel: [w262 TTL_Control."OFF" ("TTL State")] -> w259
          frame False {
          }
          frame True {
            n79 = flat-sequence {
              frame #0 {
                n80 = call "Wait3"("Count(mSec)"="HP Duration (ms)") -> ()  [unwired: 1 out]
                n81 = local write "WDW_BRK"(TRUE) -> ()
              }
              frame #1 {
                n82 = local write "WDW_BRK"(FALSE) -> ()
              }
            }
            n83 = flat-sequence {
              tunnel: [w286] -> w269
              tunnel: w269 -> [w290]
              tunnel: [w289] -> w268
              tunnel: w268 -> [w292]
              tunnel: [w292] -> w264
              frame #0 {
                n84 = call "Wait2"("Count(mSec)"="Photo Delay (ms)") -> ()  [unwired: 1 out]
              }
              frame #1 {
                w287 = TRUE
                n85 = xnode "FPGA I/O Node"("Camera TTL"=w287, "Secondary Camera TTL"=w287) -> ("error out"=w286:errorcluster)  [unwired: 3 in, 2 out]
                n86 = call "Wait4"("Count(mSec)"=u32 500) -> ()  [unwired: 1 out]
              }
              frame #2 {
                w291 = FALSE
                n87 = xnode "FPGA I/O Node"("error in"=w290, "Camera TTL"=w291, "Secondary Camera TTL"=w291) -> ("error out"=w289:errorcluster)  [unwired: 2 in, 2 out]
              }
              frame #3 {
                n88 = local write "FIRE"(FALSE) -> ()
              }
            }
            n89 = flat-sequence {
              tunnel: [w276] -> w267
              tunnel: w267 -> [w280]
              tunnel: [w279] -> w265
              frame #0 {
                n90 = call "Wait5"("Count(mSec)"="Photo 2 Delay (ms)") -> ()  [unwired: 1 out]
              }
              frame #1 {
                n91 = xnode "FPGA I/O Node"("Third Camera TTL"=TRUE) -> ("error out"=w276:errorcluster)  [unwired: 2 in, 1 out]
                n92 = call "Wait6"("Count(mSec)"=u32 500) -> ()  [unwired: 1 out]
              }
              frame #2 {
                n93 = xnode "FPGA I/O Node"("error in"=w280, "Third Camera TTL"=FALSE) -> ("error out"=w279:errorcluster)  [unwired: 1 in, 1 out]
              }
            }
            n94 = flat-sequence {
              frame #0 {
                n95 = call "Wait10"("Count(mSec)"="2nd IGN Delay (ms) 2") -> ()  [unwired: 1 out]
              }
              frame #1 {
                n96 = local write "2nd_IGN"(TRUE ("2nd_IGN")) -> ()
                n97 = call "Wait11"("Count(mSec)"=u32 5000) -> ()  [unwired: 1 out]
              }
              frame #2 {
                n98 = local write "2nd_IGN"(FALSE ("2nd_IGN")) -> ()
              }
            }
            n99 = Merge Errors(w264, w265) -> (w263:errorcluster)
            n100 = Unbundle By Name(w263) -> ("status"=→"9401 Fault":bool)
          }
        }
      }
      frame "OFF", Default {
        w296 = FALSE
        n101 = xnode "FPGA I/O Node"("Spectrometer TTL"=w296, "Camera TTL"=w296, "Secondary Camera TTL"=w296, "Ignitor"=w296, "9401_WDW_BRK"=w296, "Grill"=w296) -> ()  [unwired: 7 in, 7 out]
        n102 = local write "WDW_BRK"(FALSE) -> ()
        n103 = local write "2nd_IGN"(FALSE ("2nd_IGN")) -> ()
      }
      frame "MANUAL" {
      }
    }
    n104 = Equal?(x="TTL State", y=w256) -> (x = y?=w257:bool)
    n105 = Select(t=w256, s=w257, f="TTL State") -> (s? t:f=w254:T11)
  }
  n106 = while {
    shift-right: [w359] -> _
    shift-left: _ -> [w352]
    shift-right: [w358] -> _
    shift-left: _ -> [w351]
    shift-right: [w357] -> _
    shift-left: _ -> [w350]
    shift-right: [w356] -> _
    shift-left: _ -> [w349]
    shift-right: [w355] -> _
    shift-left: _ -> [w348]
    shift-right: [w354] -> _
    shift-left: _ -> [w347]
    shift-right: [w353] -> _
    shift-left: _ -> [w346]
    shift-right: [w345] -> _
    shift-left: _ -> [w344]
    shift-right: [w343] -> _
    shift-left: _ -> [w341]
    shift-right: [w342] -> _
    shift-left: _ -> [w340]
    shift-right: [w339] -> _
    shift-left: _ -> [w338]
    shift-right: [w337] -> _
    shift-left: _ -> [w335]
    shift-right: [w336] -> _
    shift-left: _ -> [w334]
    shift-right: [w333] -> _
    shift-left: _ -> [w329]
    shift-right: [w332] -> _
    shift-left: _ -> [w328]
    shift-right: [w331] -> _
    shift-left: _ -> [w327]
    shift-right: [w330] -> _
    shift-left: _ -> [w326]
    shift-right: [w325] -> _
    shift-left: _ -> [w322]
    shift-right: [w324] -> _
    shift-left: _ -> [w321]
    shift-right: [w323] -> _
    shift-left: _ -> [w320]
    stop <- FALSE stop-if-true
    # "Monitoring Loop"
    n107 = flat-sequence {
      tunnel: w320 -> [w362]
      tunnel: w321 -> [w363]
      tunnel: w322 -> [w364]
      tunnel: w326 -> [w365]
      tunnel: w327 -> [w366]
      tunnel: w328 -> [w367]
      tunnel: w329 -> [w368]
      tunnel: w334 -> [w369]
      tunnel: w335 -> [w370]
      tunnel: w338 -> [w371]
      tunnel: w340 -> [w372]
      tunnel: w341 -> [w373]
      tunnel: w344 -> [w374]
      tunnel: w346 -> [w375]
      tunnel: w347 -> [w376]
      tunnel: w348 -> [w377]
      tunnel: w349 -> [w378]
      tunnel: w350 -> [w379]
      tunnel: w351 -> [w380]
      tunnel: w352 -> [w381]
      tunnel: [w381] -> w319
      tunnel: [w380] -> w318
      tunnel: [w379] -> w317
      tunnel: [w378] -> w316
      tunnel: [w377] -> w315
      tunnel: [w376] -> w314
      tunnel: [w375] -> w313
      tunnel: [w374] -> w312
      tunnel: [w373] -> w311
      tunnel: [w372] -> w310
      tunnel: [w371] -> w309
      tunnel: [w370] -> w308
      tunnel: [w369] -> w307
      tunnel: [w368] -> w306
      tunnel: [w367] -> w305
      tunnel: [w366] -> w304
      tunnel: [w365] -> w303
      tunnel: [w364] -> w302
      tunnel: [w363] -> w301
      tunnel: [w362] -> w300
      tunnel: [w463] -> w359
      tunnel: [w462] -> w358
      tunnel: [w461] -> w357
      tunnel: [w460] -> w356
      tunnel: [w459] -> w355
      tunnel: [w458] -> w354
      tunnel: [w457] -> w353
      tunnel: [w433] -> w345
      tunnel: [w430] -> w343
      tunnel: [w429] -> w342
      tunnel: [w422] -> w339
      tunnel: [w416] -> w337
      tunnel: [w415] -> w336
      tunnel: [w410] -> w333
      tunnel: [w409] -> w332
      tunnel: [w408] -> w331
      tunnel: [w407] -> w330
      tunnel: [w394] -> w325
      tunnel: [w393] -> w324
      tunnel: [w392] -> w323
      tunnel: w319 -> [w456]
      tunnel: w318 -> [w455]
      tunnel: w317 -> [w454]
      tunnel: w316 -> [w453]
      tunnel: w315 -> [w452]
      tunnel: w314 -> [w451]
      tunnel: w313 -> [w450]
      tunnel: w312 -> [w432]
      tunnel: w311 -> [w428]
      tunnel: w310 -> [w427]
      tunnel: w309 -> [w421]
      tunnel: w308 -> [w414]
      tunnel: w307 -> [w413]
      tunnel: w306 -> [w406]
      tunnel: w305 -> [w404]
      tunnel: w304 -> [w403]
      tunnel: w303 -> [w402]
      tunnel: w302 -> [w388]
      tunnel: w301 -> [w387]
      tunnel: w300 -> [w386]
      frame #0 {
        n108 = call "Loop Timer"("Count(mSec)"=u32 50) -> ("Tick Count(mSec)"=→"Tick Count(mSec)":u32)
      }
      frame #1 {
        w446 = T4 {"LOX_TANK_ULEGE"=0.0, "LNG_DIFF"=0.0, "LOX_DIFF"=0.0, "LOX_TANK 2"=0.0, "LNG_TANK 2"=0.0, "LOX_TANK_ULEGE 2"=0.0, "LNG_TANK_ULEGE"=0.0, "LNG_TANK_ULEGE 2"=0.0}  # IN TANK MEASUREMENTS
        w445 = T3 {"LNG_DST"=0.0, "LNG_DSP"=0.0, "LOX_DST"=0.0, "LOX_DSP"=0.0, "N2_PURGE [CFM]"=0.0, "LNG_USP"=0.0, "LOX_USP "=0.0, "LNG_UST"=0.0, "LOX_UST"=0.0, "LNG_MST"=0.0, "LNG_MSP"=0.0, "LOX_MST\n"=0.0, "LOX_MSP"=0.0, "LOX_DST 2"=0.0, "LNG_DST 2"=0.0, "LN2_Temp_HEX"=0.0, "LN2_Temp_Coil"=0.0, "LN2 [GPM]"=0.0}  # SYSTEM MEASUREMENTS
        n109 = xnode "Mean, Variance, and Standard Deviation"("input data"=w452) -> ("mean"=w466:fxp<+/-,26,5>)  [unwired: 1 in, 1 out]
        n110 = xnode "Mean, Variance, and Standard Deviation"("input data"=w451) -> ("mean"=w465:fxp<+/-,26,5>)  [unwired: 1 in, 1 out]
        n111 = xnode "Mean, Variance, and Standard Deviation"("input data"=w450) -> ("mean"=w464:fxp<+/-,26,5>)  [unwired: 1 in, 1 out]
        n112 = xnode "Mean, Variance, and Standard Deviation"("input data"=w414) -> ("mean"=w418:fxp<+/-,26,5>)  [unwired: 1 in, 1 out]
        n113 = xnode "Mean, Variance, and Standard Deviation"("input data"=w413) -> ("mean"=w417:fxp<+/-,26,5>)  [unwired: 1 in, 1 out]
        n114 = xnode "Mean, Variance, and Standard Deviation"("input data"=w428) -> ("mean"=w425:fxp<+/-,26,5>)  [unwired: 1 in, 1 out]
        n115 = xnode "Mean, Variance, and Standard Deviation"("input data"=w427) -> ("mean"=w426:fxp<+/-,26,5>)  [unwired: 1 in, 1 out]
        n116 = xnode "Mean, Variance, and Standard Deviation"("input data"=w421) -> ("mean"=w420:fxp<+/-,26,5>)  [unwired: 1 in, 1 out]
        n117 = To Single Precision Float(number=w418) -> (single precision float=w412:sgl)
        n118 = To Single Precision Float(number=w417) -> (single precision float=w411:sgl)
        n119 = To Single Precision Float(number=w425) -> (single precision float=w424:sgl)
        n120 = xnode "Mean, Variance, and Standard Deviation"("input data"=w406) -> ("mean"=w405:fxp<+/-,26,5>)  [unwired: 1 in, 1 out]
        n121 = To Single Precision Float(number=w426) -> (single precision float=w423:sgl)
        n122 = To Single Precision Float(number=w420) -> (single precision float=w419:sgl)
        n123 = xnode "Mean, Variance, and Standard Deviation"("input data"=w404) -> ("mean"=w401:fxp<+/-,26,5>)  [unwired: 1 in, 1 out]
        n124 = xnode "Mean, Variance, and Standard Deviation"("input data"=w403) -> ("mean"=w400:fxp<+/-,26,5>)  [unwired: 1 in, 1 out]
        n125 = To Single Precision Float(number=w466) -> (single precision float=w448:sgl)
        "LNG_DIFF" <- w448
        n126 = To Single Precision Float(number=w465) -> (single precision float=w449:sgl)
        "LOX_DIFF" <- w449
        n127 = To Single Precision Float(number=w464) -> (single precision float=w443:sgl)
        "LOX_UP" <- w443
        n128 = xnode "Mean, Variance, and Standard Deviation"("input data"=w388) -> ("mean"=w391:fxp<+/-,24,5>)  [unwired: 1 in, 1 out]
        n129 = xnode "Mean, Variance, and Standard Deviation"("input data"=w387) -> ("mean"=w390:fxp<+/-,24,5>)  [unwired: 1 in, 1 out]
        n130 = xnode "Mean, Variance, and Standard Deviation"("input data"=w402) -> ("mean"=w399:fxp<+/-,26,5>)  [unwired: 1 in, 1 out]
        n131 = xnode "Mean, Variance, and Standard Deviation"("input data"=w386) -> ("mean"=w389:fxp<+/-,24,5>)  [unwired: 1 in, 1 out]
        n132 = xnode "Mean, Variance, and Standard Deviation"("input data"=w455) -> ("mean"=w439:fxp<+/-,26,5>)  [unwired: 1 in, 1 out]
        n133 = xnode "Mean, Variance, and Standard Deviation"("input data"=w454) -> ("mean"=w437:fxp<+/-,26,5>)  [unwired: 1 in, 1 out]
        n134 = xnode "Mean, Variance, and Standard Deviation"("input data"=w453) -> ("mean"=w435:fxp<+/-,26,5>)  [unwired: 1 in, 1 out]
        n135 = xnode "Mean, Variance, and Standard Deviation"("input data"=w432) -> ("mean"=w431:fxp<+/-,26,5>)  [unwired: 1 in, 1 out]
        n136 = xnode "Mean, Variance, and Standard Deviation"("input data"=w456) -> ("mean"=w441:fxp<+/-,26,5>)  [unwired: 1 in, 1 out]
        n137 = To Single Precision Float(number=w405) -> (single precision float=w398:sgl)
        n138 = To Single Precision Float(number=w400) -> (single precision float=w396:sgl)
        n139 = To Single Precision Float(number=w399) -> (single precision float=w395:sgl)
        n140 = To Single Precision Float(number=w401) -> (single precision float=w397:sgl)
        n141 = To Single Precision Float(number=w391) -> (single precision float=w384:sgl)
        n142 = To Single Precision Float(number=w390) -> (single precision float=w383:sgl)
        n143 = To Single Precision Float(number=w389) -> (single precision float=w382:sgl)
        n144 = To Single Precision Float(number=w441) -> (single precision float=w440:sgl)
        "LNG_DST" <- w440
        n145 = To Single Precision Float(number=w439) -> (single precision float=w438:sgl)
        "LOX_DST" <- w438
        n146 = To Single Precision Float(number=w437) -> (single precision float=w436:sgl)
        "LNG_DSP" <- w436
        n147 = To Single Precision Float(number=w435) -> (single precision float=w434:sgl)
        "LOX_DSP" <- w434
        n148 = To Single Precision Float(number=w431) -> (single precision float=w385:sgl)
        "N2F" <- w385
        n149 = Bundle By Name(cluster=w446, "LNG_DIFF"=w448, "LOX_DIFF"=w449, "LOX_TANK_ULEGE"=w443, "LNG_TANK 2"=w424, "LOX_TANK 2"=w423, "LOX_TANK_ULEGE 2"=w419, "LNG_TANK_ULEGE"=w412, "LNG_TANK_ULEGE 2"=w411) -> (→"IN TANK MEASUREMENTS":T4)
        n150 = Bundle By Name(cluster=w445, "N2_PURGE [CFM]"=w385, "LNG_DST"=w440, "LOX_DST"=w438, "LNG_DSP"=w436, "LOX_DSP"=w434, "LNG_USP"=w398, "LOX_USP"=w397, "LNG_MSP"=w396, "LOX_MSP"=w395, "LN2_Temp_HEX"=w384, "LN2_Temp_Coil"=w382, "LN2 [GPM]"=w383) -> (→"SYSTEM MEASUREMENTS":T3)
        n151 = xnode "FPGA I/O Node"() -> ("Mod7/AI0/LN2_Temp_HE"=w394:fxp<+/-,24,5>, "Mod7/AI1/LNG_FR"=w393:fxp<+/-,24,5>, "Mod7/AI2/N2_Coil_Temp"=w392:fxp<+/-,24,5>)  [unwired: 3 in, 3 out]
        n152 = xnode "FPGA I/O Node"() -> ("error out"=→"error out":errorcluster, "Mod4/AI6/LNG_DST"=w463:fxp<+/-,26,5>, "Mod4/AI7/LOX_DST"=w462:fxp<+/-,26,5>, "Mod4/AI18/LNG_DSP"=w461:fxp<+/-,26,5>, "Mod4/AI19/LOX_DSP"=w460:fxp<+/-,26,5>, "Mod4/AI16/LNG_DIFF"=w459:fxp<+/-,26,5>, "Mod4/AI17/LOX_DIFF"=w458:fxp<+/-,26,5>, "Mod4/AI12/LOX_UP"=w457:fxp<+/-,26,5>, "Mod4/AI23/N2F"=w433:fxp<+/-,26,5>, "Mod4/AI8/LNG_THP2"=w430:fxp<+/-,26,5>, "Mod4/AI9/LOX_THP2"=w429:fxp<+/-,26,5>, "Mod4/AI13/LOX_UP2"=w422:fxp<+/-,26,5>, "Mod4/AI0/LNG_UP"=w416:fxp<+/-,26,5>, "Mod4/AI1/LNG_UP2"=w415:fxp<+/-,26,5>, "Mod4/AI20/LNG_USP"=w410:fxp<+/-,26,5>, "Mod4/AI21/LOX_USP"=w409:fxp<+/-,26,5>, "Mod4/AI28/LOX_MSP"=w408:fxp<+/-,26,5>, "Mod4/AI31/LNG_MSP"=w407:fxp<+/-,26,5>)  [unwired: 18 in, 17 out]
        "Mod4/AI6/LNG_DST" <- w463
      }
    }
  }
  n153 = while {
    shift-right: [w2005] -> _
    shift-left: _ -> [w1999]
    shift-right: [w2004] -> _
    shift-left: _ -> [w1997]
    shift-right: [w2003] -> _
    shift-left: _ -> [w1995]
    shift-right: [w2002] -> _
    shift-left: _ -> [w1993]
    shift-right: [w2001] -> _
    shift-left: _ -> [w1991]
    shift-right: [w2000] -> _
    shift-left: _ -> [w1989]
    stop <- FALSE stop-if-true
    n154 = flat-sequence {
      tunnel: w1999 -> [w2011]
      tunnel: [w2011] -> w1998
      tunnel: w1997 -> [w2010]
      tunnel: [w2010] -> w1996
      tunnel: w1995 -> [w2009]
      tunnel: [w2009] -> w1994
      tunnel: w1993 -> [w2008]
      tunnel: [w2008] -> w1992
      tunnel: w1991 -> [w2007]
      tunnel: [w2007] -> w1990
      tunnel: w1989 -> [w2006]
      tunnel: [w2006] -> w1988
      tunnel: [w2039] -> w2005
      tunnel: [w2038] -> w2004
      tunnel: [w2037] -> w2003
      tunnel: [w2036] -> w2002
      tunnel: [w2035] -> w2001
      tunnel: [w2034] -> w2000
      tunnel: w1998 -> [w2018]
      tunnel: w1996 -> [w2017]
      tunnel: w1994 -> [w2016]
      tunnel: w1992 -> [w2015]
      tunnel: w1990 -> [w2014]
      tunnel: w1988 -> [w2013]
      frame #0 {
        n155 = call "Loop Timer2"("Count(mSec)"=u32 100) -> ()  [unwired: 1 out]
      }
      frame #1 {
        n156 = xnode "Mean, Variance, and Standard Deviation"("input data"=w2018) -> ("mean"=w2028:fxp<+/-,24,-4>)  [unwired: 1 in, 1 out]
        n157 = xnode "Mean, Variance, and Standard Deviation"("input data"=w2017) -> ("mean"=w2029:fxp<+/-,24,-4>)  [unwired: 1 in, 1 out]
        n158 = xnode "Mean, Variance, and Standard Deviation"("input data"=w2016) -> ("mean"=w2030:fxp<+/-,24,-4>)  [unwired: 1 in, 1 out]
        n159 = xnode "Mean, Variance, and Standard Deviation"("input data"=w2015) -> ("mean"=w2031:fxp<+/-,24,-4>)  [unwired: 1 in, 1 out]
        n160 = xnode "Mean, Variance, and Standard Deviation"("input data"=w2014) -> ("mean"=w2032:fxp<+/-,24,-4>)  [unwired: 1 in, 1 out]
        n161 = xnode "Mean, Variance, and Standard Deviation"("input data"=w2013) -> ("mean"=w2033:fxp<+/-,24,-4>)  [unwired: 1 in, 1 out]
        n162 = To Single Precision Float(number=w2028) -> (single precision float=w2019:sgl)
        "LNG_FMF" <- w2019
        n163 = To Single Precision Float(number=w2029) -> (single precision float=w2020:sgl)
        "LNG_FMT" <- w2020
        n164 = To Single Precision Float(number=w2030) -> (single precision float=w2021:sgl)
        "LNG_FMP" <- w2021
        n165 = To Single Precision Float(number=w2031) -> (single precision float=w2022:sgl)
        "LOX_FMF" <- w2022
        n166 = To Single Precision Float(number=w2032) -> (single precision float=w2023:sgl)
        "LOX_FMT" <- w2023
        n167 = To Single Precision Float(number=w2033) -> (single precision float=w2024:sgl)
        "LOX_FMP" <- w2024
        n168 = Bundle By Name(cluster=T2 {"LNG_FMT [F]"=0.0, "LOX_FMT [F]"=0.0, "LOX_FMP [psi]"=0.0, "LNG_FMP [psi]"=0.0, "LOX_FMF [GPM]"=0.0, "LNG_FMF [GPM]"=0.0} ("FM Indicators 2"), "LNG_FMF [GPM]"=w2019, "LNG_FMT [F]"=w2020, "LNG_FMP [psi]"=w2021, "LOX_FMF [GPM]"=w2022, "LOX_FMT [F]"=w2023, "LOX_FMP [psi]"=w2024) -> (→"FM Indicators":T2)
        n169 = xnode "FPGA I/O Node"() -> ("error out"=→"error out 2":errorcluster, "FQ-02 (LNG_FMF)"=w2039:fxp<+/-,24,-4>, "TI-07 (LNG_FMT)"=w2038:fxp<+/-,24,-4>, "PT-16 (LNG_FMP)"=w2037:fxp<+/-,24,-4>, "FQ-01 (LOX_FMF)"=w2036:fxp<+/-,24,-4>, "TI-02 (LOX_FMT)"=w2035:fxp<+/-,24,-4>, "PT-06 (LOX_FMP)"=w2034:fxp<+/-,24,-4>)  [unwired: 7 in, 6 out]
      }
    }
  }
  n170 = Add(x=u8 11 ("IRQ Number (0)"), y=u8 11 ("IRQ Number (0)")) -> (x+y=→"x+y 4":u8)
